vi "increasing and decreasing using glo56ba66+.vi"() -> ()   [LabVIEW 2018]
panel:
  out "Slide":dbl(slide) scale=0.0..10.0
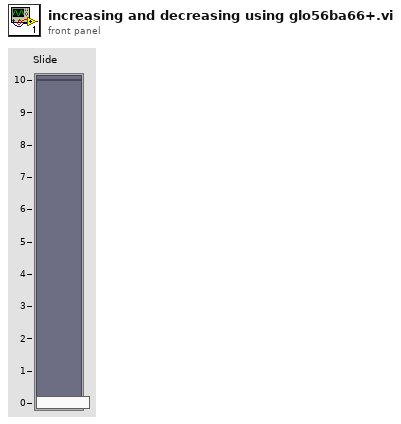
[diagram p1: front panel]
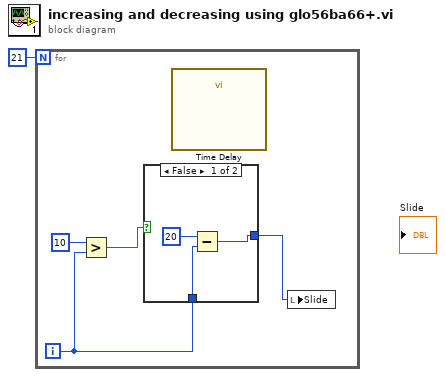
[diagram p0: block diagram]
diagram:
  n1 = for {
    N: 21 -> [_]
    i -> [w3]
    n2 = Greater?(x=10, y=w3) -> (0:w4:bool)
    n3 = case shown="False" w4 {
      tunnel: w3 -> [w8 w9]
      tunnel: [w6 w9] -> w2
      frame False {
        n4 = Subtract(x=20, y=w8) -> (x-y=w6:i32)
      }
      frame True {
      }
    }
    n5 = call "Time Delay"() -> ()  [unwired: 11 in, 1 out]
    n6 = local write "Slide"(w2) -> ()
  }
